vi "Station Get New.vi"(8 "error in (no error)":errorcluster, 11 "Connection Refnum":T1) -> (0 "error out":errorcluster, 1 "Instruments on Station":T2[](array[typedef]), 2 "New Test Station":T3, 3 "Connection Refnum":T1)   [LabVIEW 2011]
uses:
  Station Record.ctl
  Instruments/Instrument Record.ctl
  SI.LIB/ODBC/SQL Controls/Connection Refnum.ctl
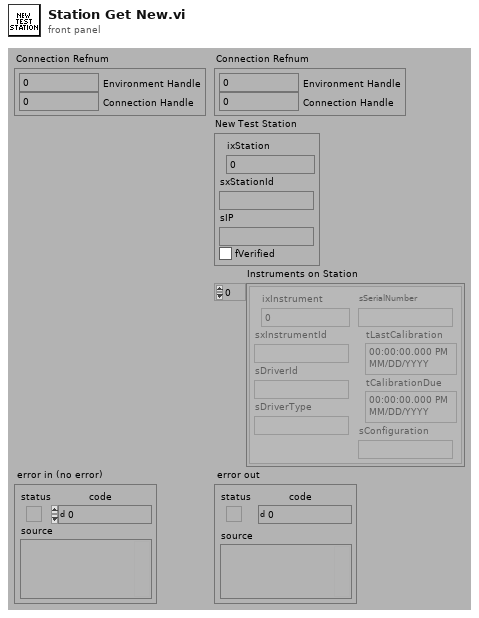
[diagram p1: front panel]
types:
  T1 = typedef "Connection Refnum.ctl" = cluster{"Environment Handle":i32, "Connection Handle":i32}
  T2 = typedef "Instrument Record.ctl" = cluster{"ixInstrument":i32, "sxInstrumentId":string, "sDriverId":string, "sDriverType":string, "sSerialNumber":string, "tLastCalibration":timestamp, "tCalibrationDue":timestamp, "sConfiguration":string}
  T3 = typedef "Station Record.ctl" = cluster{"ixStation":i32, "sxStationId":string, "sIP":string, "fVerified":bool}
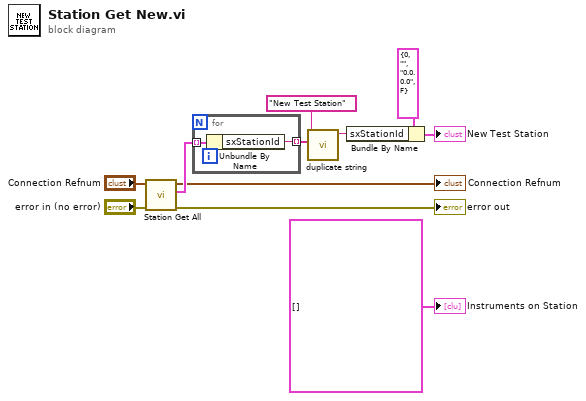
[diagram p0: block diagram]
diagram:
  n1 = call "Station Get All.vi"("error in (no error)"="error in (no error)", "Connection Refnum"="Connection Refnum") -> ("error out"=→"error out":errorcluster, "Station Records"=w5:T3[], "Connection Refnum"=→"Connection Refnum":T1)  [unwired: 2 in, 5 out]
  n2 = for {
    tunnel: w5 -> [w13] mode=indexing
    tunnel: [w12] -> w10 mode=indexing
    n3 = Unbundle By Name(w13) -> ("sxStationId"=w12:string)
  }
  n4 = call "duplicate string.vi"("Array of Strings"=w10, "String"="New Test Station") -> ("Updated String"=w7:string)  [unwired: 9 out]
  n5 = Bundle By Name(cluster=T3 {"ixStation"=0, "sxStationId"="", "sIP"="0.0.0.0", "fVerified"=FALSE} ("Default New User"), "sxStationId"=w7) -> (→"New Test Station":T3)
  "Instruments on Station" <- T2[] [] ("Instruments on Station")
